vi "采配水PLC通讯.vi"() -> ()   [LabVIEW 2016, in "PLC.lvlib"]
uses:
  PLC.lvlib
  <vilib>/Plasmionique/MB Master/MB_Master/MB_Master.lvclass
  <vilib>/Plasmionique/MB Master/MB_Master_Serial/MB_Master_Serial.lvclass
  D:/Program Files (x86)/National Instruments/LabVIEW 2016/vi.lib/Plasmionique/MB Master/MB_Master/MB_Master.lvclass
  <vilib>/Plasmionique/MB Master/MB Master.lvlib
panel:
  in  "单个写入参数":T1
  in  "单个写入":bool
  in  "多个写入参数":T2
  in  "多个写入":bool
  out "元素":cluster{"命令":string, "数据":variant}[](array[cluster])
  out "待处理插入数量":i32
  out "待处理删除数量":i32
  out "队列中元素数量":i32
  in  "读状态":bool
  out "命令":string
  in  "停止":bool
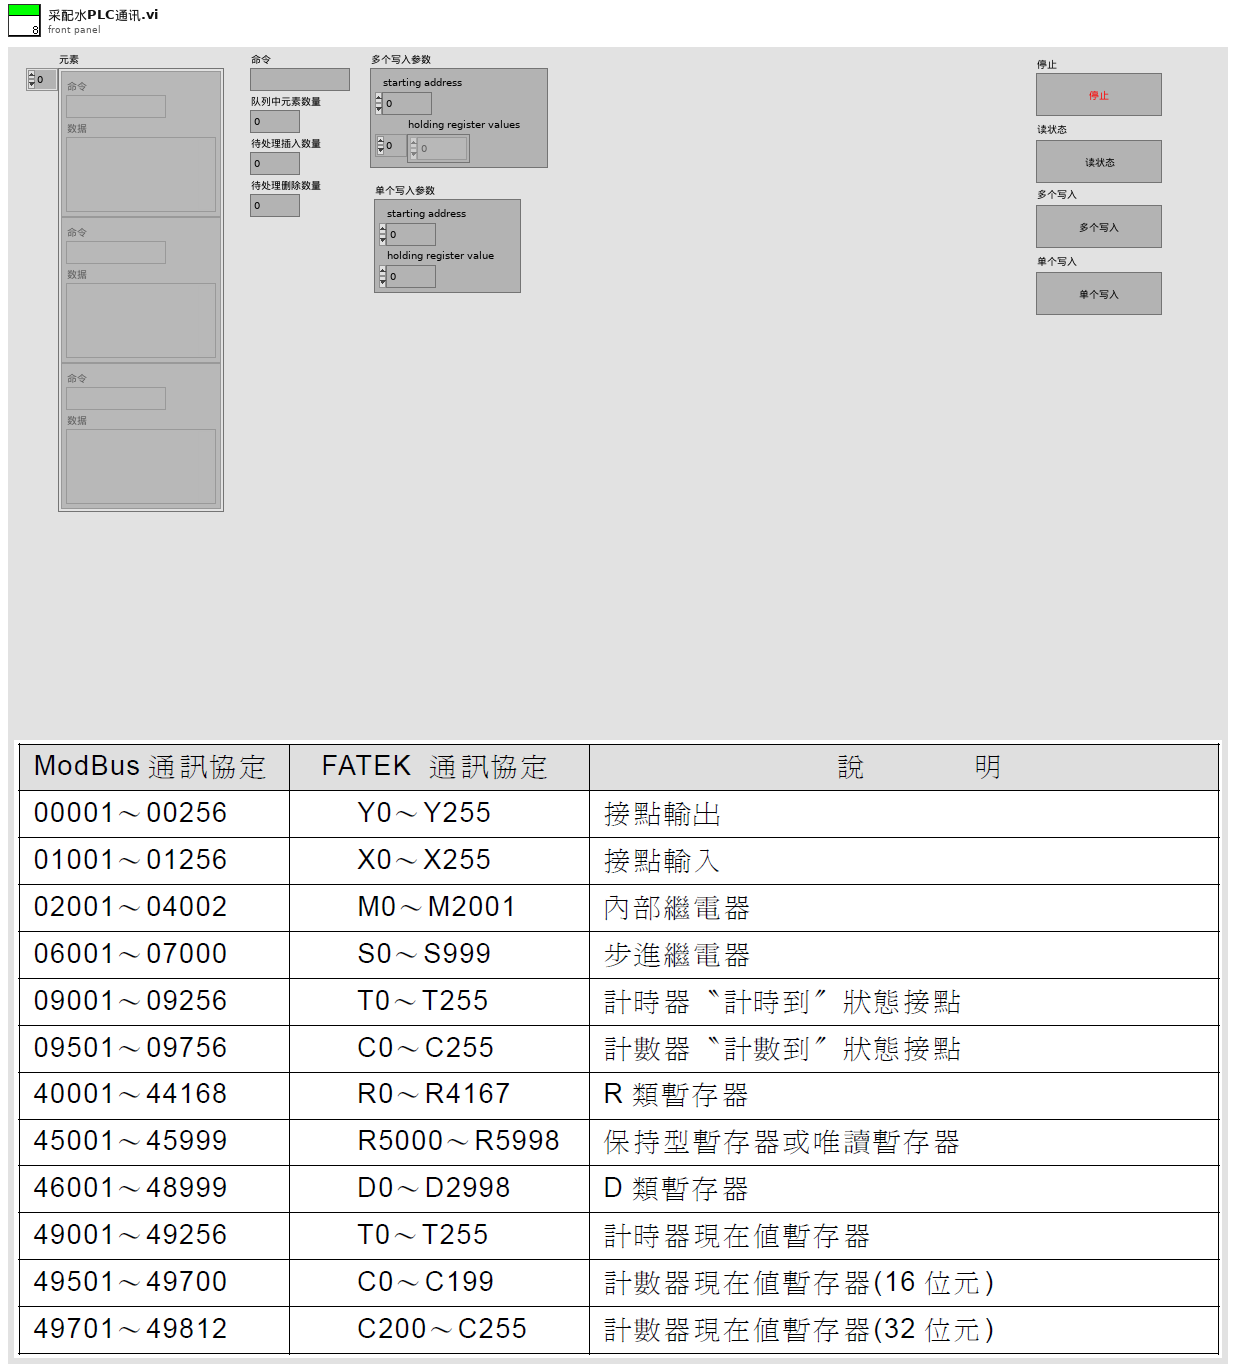
[diagram p1: front panel]
types:
  T1 = cluster{"starting address":u16, "holding register value":u16}
  T2 = cluster{"starting address":u16, "holding register values":u16[]}
  T3 = cluster{"baud rate (bps)":u32, "stop bits":u16, "parity":u16, "flow control":u16, "timeout":u32, "retries":i32}
  T4 = cluster{"starting address":u16, "coil values":bool[]}
  T5 = cluster{"Registers[0]":u16, "Registers[1]":u16, "Registers[2]":u16, "Registers[3]":u16, "Registers[4]":u16, "Registers[5]":u16, "Registers[6]":u16, "Registers[7]":u16, "Registers[8]":u16, "Registers[9]":u16, "Registers[10]":u16, "Registers[11]":u16, "Registers[12]":u16, "Registers[13]":u16, "Registers[14]":u16, "Registers[15]":u16, "Registers[16]":u16, "Registers[17]":u16, "Registers[18]":u16, "Registers[19]":u16}
  T6 = cluster{"Registers[0]":u16, "Registers[1]":u16, "Registers[2]":u16, "Registers[3]":u16, "Registers[4]":u16, "Registers[5]":u16}
  T7 = cluster{"Coils[0]":bool, "Coils[1]":bool, "Coils[2]":bool, "Coils[3]":bool, "Coils[4]":bool, "Coils[5]":bool, "Coils[6]":bool, "Coils[7]":bool, "Coils[8]":bool, "Coils[9]":bool, "Coils[10]":bool, "Coils[11]":bool, "Coils[12]":bool, "Coils[13]":bool, "Coils[14]":bool, "Coils[15]":bool}
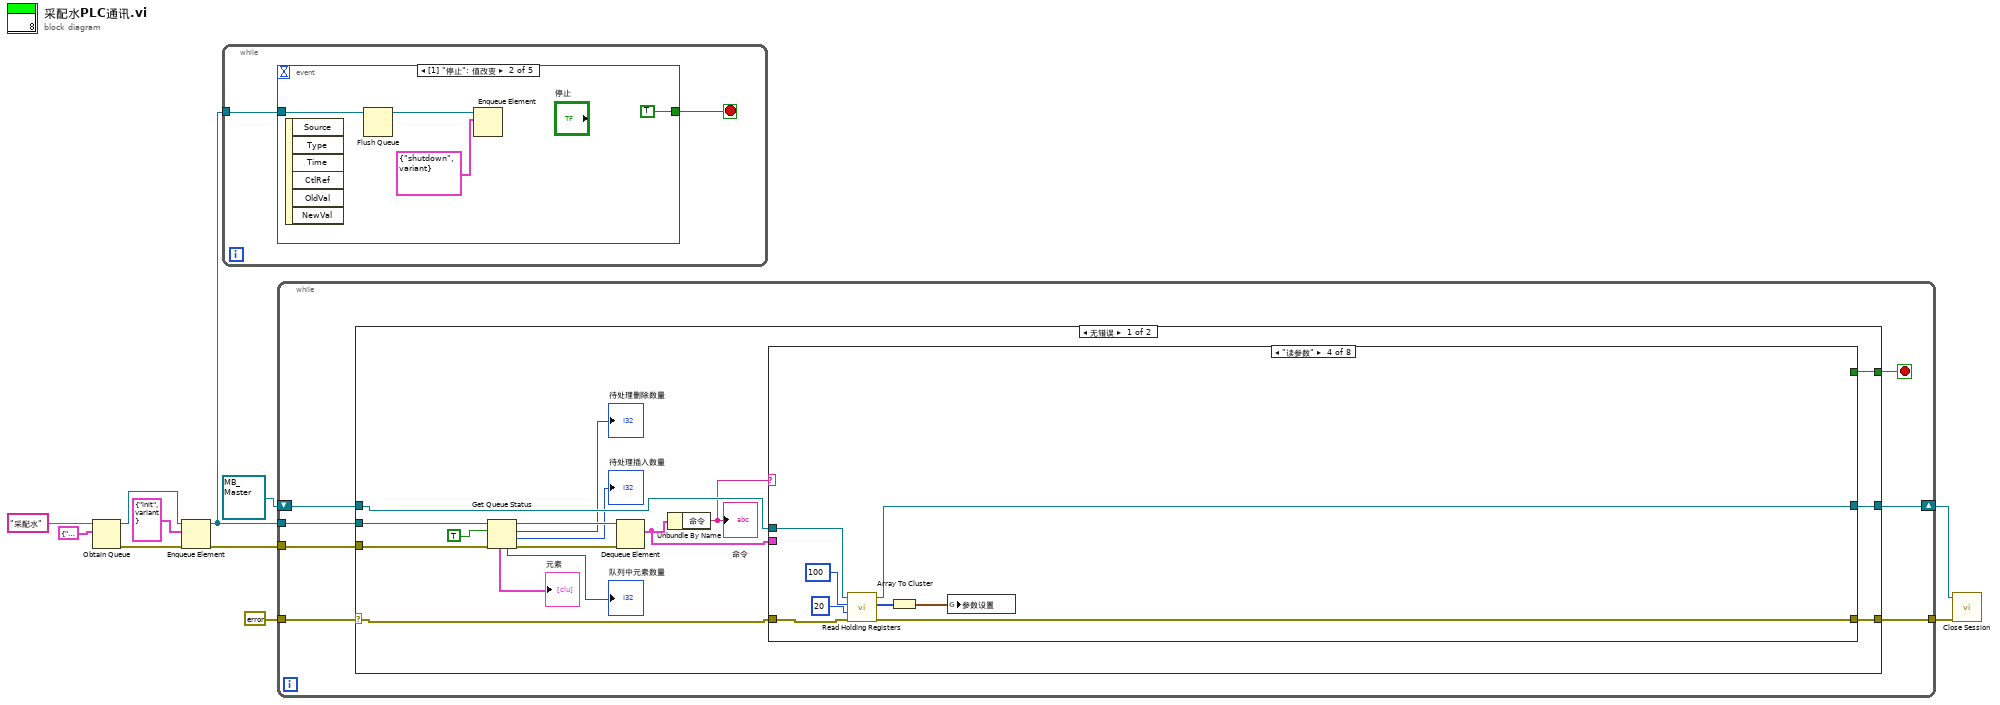
[diagram p0: block diagram]
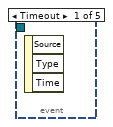
[diagram p2: hidden frame]
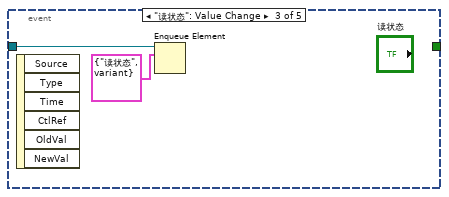
[diagram p3: hidden frame]
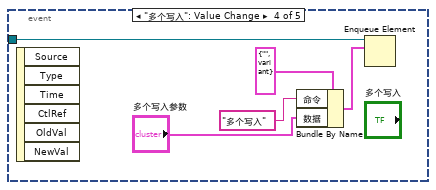
[diagram p4: hidden frame]
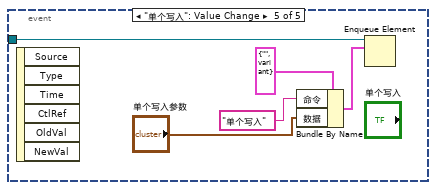
[diagram p5: hidden frame]
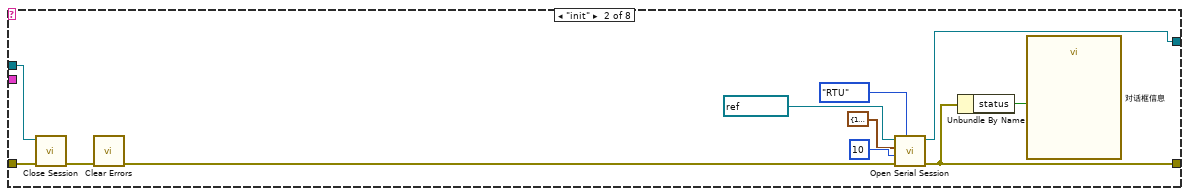
[diagram p7: hidden frame]
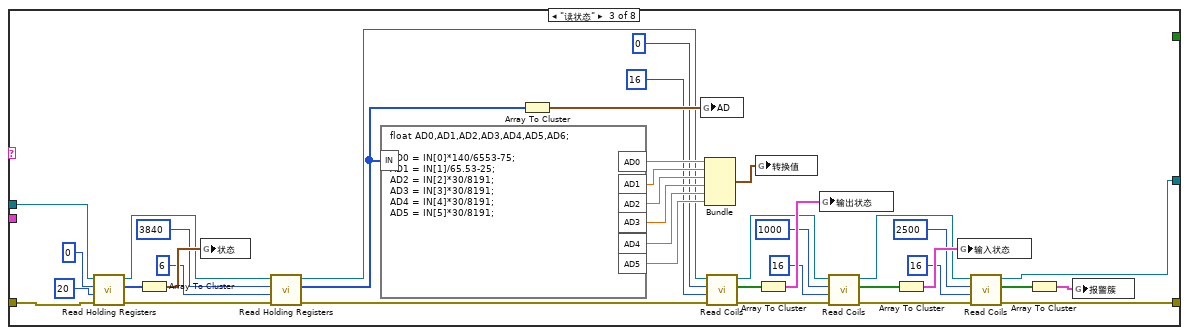
[diagram p8: hidden frame]
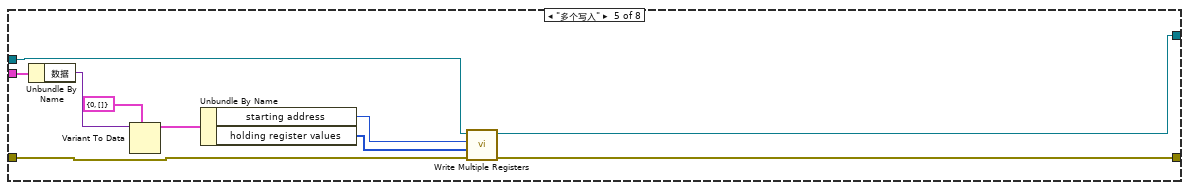
[diagram p9: hidden frame]
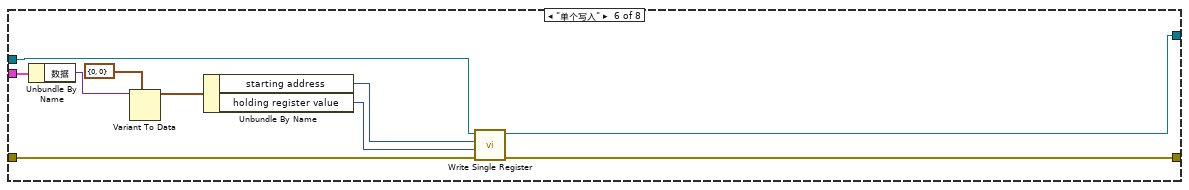
[diagram p10: hidden frame]
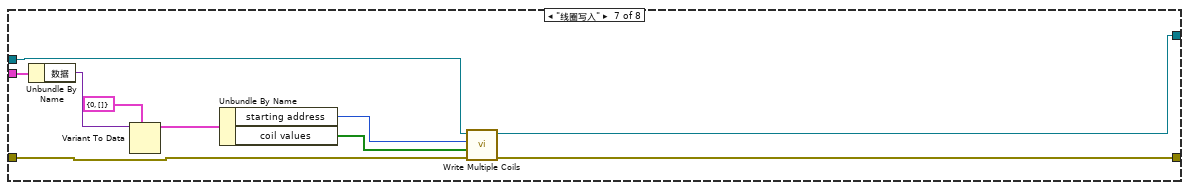
[diagram p11: hidden frame]
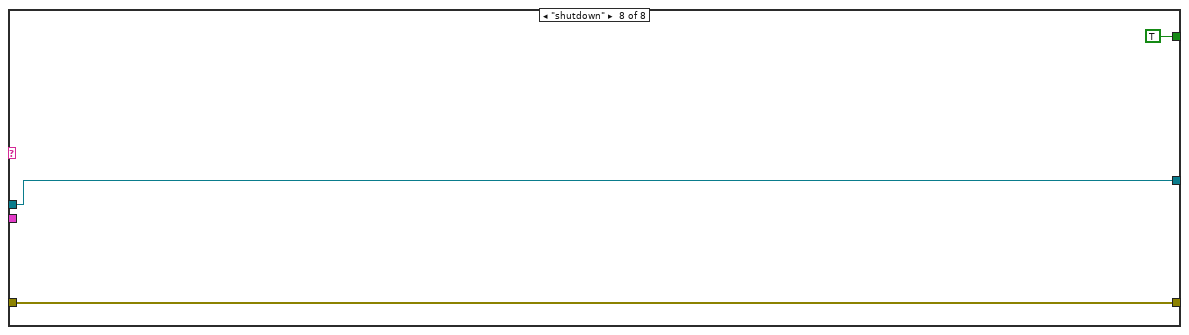
[diagram p12: hidden frame]
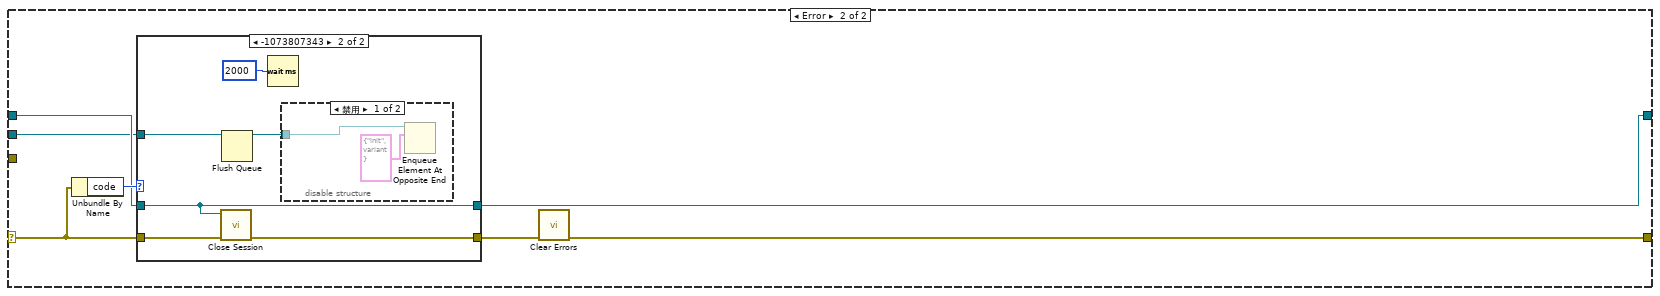
[diagram p13: hidden frame]
diagram:
  n1 = Obtain Queue(name (unnamed)="采配水" ("名称（未命名）"), element data type=cluster{"命令":string, "数据":variant} {"命令"="", "数据"=variant}) -> (queue out=w9:refnum<queue>, error out=w8:errorcluster)  [unwired: 3 in, 1 out]
  n2 = Enqueue Element(queue=w9, element=cluster{"命令":string, "数据":variant} {"命令"="init", "数据"=variant} ("元素"), error in (no error)=w8) -> (queue out=w4:refnum<queue>, error out=w6:errorcluster)  [unwired: 1 in, 1 out]
  n3 = while {
    tunnel: w4 -> [w13]
    stop <- w12 stop-if-true
    n4 = event shown="[1] \"停止\": 值改变" {
      selector: _ -> [_ _ _ _ _]
      dyn-events: _ -> [_ _ _ _ _]
      timeout: _ -> [_ _ _ _ _]
      tunnel: w13 -> [_ w16 w19 w24 w29]
      tunnel: [_ TRUE _ _ _] -> w12
      event Timeout {
        n5 = event-data() -> ()  [unwired: 1 in, 3 out]
      }
      event "停止": Value Change {
        n6 = event-data() -> ()  [unwired: 1 in, 6 out]
        n7 = Flush Queue(queue=w16) -> (queue out=w14:refnum<queue>)  [unwired: 1 in, 2 out]
        n8 = Enqueue Element(queue=w14, element=cluster{"命令":string, "数据":variant} {"命令"="shutdown", "数据"=variant} ("元素")) -> ()  [unwired: 2 in, 3 out]
      }
      event "读状态": Value Change {
        n9 = event-data() -> ()  [unwired: 1 in, 6 out]
        n10 = Enqueue Element(queue=w19, element=cluster{"命令":string, "数据":variant} {"命令"="读状态", "数据"=variant} ("元素")) -> ()  [unwired: 2 in, 3 out]
      }
      event "多个写入": Value Change {
        n11 = event-data() -> ()  [unwired: 1 in, 6 out]
        n12 = Bundle By Name(cluster=cluster{"命令":string, "数据":variant} {"命令"="", "数据"=variant} ("元素"), "命令"="多个写入", "数据"="多个写入参数") -> (w20:cluster{"命令":string, "数据":variant})
        n13 = Enqueue Element(queue=w24, element=w20) -> ()  [unwired: 2 in, 3 out]
      }
      event "单个写入": Value Change {
        n14 = event-data() -> ()  [unwired: 1 in, 6 out]
        n15 = Bundle By Name(cluster=cluster{"命令":string, "数据":variant} {"命令"="", "数据"=variant} ("元素"), "命令"="单个写入", "数据"="单个写入参数") -> (w26:cluster{"命令":string, "数据":variant})
        n16 = Enqueue Element(queue=w29, element=w26) -> ()  [unwired: 2 in, 3 out]
      }
    }
  }
  n17 = while {
    tunnel: w4 -> [w32]
    tunnel: w6 -> [w31]
    shift-right: [w36] -> w1
    shift-left: refnum<class "MB_Master.lvclass"> refnum ("MB session in") -> [w35]
    tunnel: errorcluster {"status"=FALSE, "code"=0, "source"=""} ("error out") -> [w33]
    tunnel: [w34] -> w2
    stop <- w30 stop-if-true
    n18 = case shown="无错误" w33 {
      selector: w33 -> [w49 w150]
      tunnel: [w52 w149] -> w36
      tunnel: w35 -> [w51 w151]
      tunnel: [w50 w147] -> w34
      tunnel: w32 -> [w46 w146]
      tunnel: w31 -> [w45 _]
      tunnel: [w47 _] -> w30
      frame No Error {
        n19 = Get Queue Status(queue=w46, return elements? (F)=TRUE ("返回元素？(F)"), error in (no error)=w45) -> (queue out=w44:refnum<queue>, # pending remove=→"待处理删除数量":i32, # pending insert=→"待处理插入数量":i32, error out=w43:errorcluster, # elements in queue=→"队列中元素数量":i32, elements=→"元素":cluster{"命令":string, "数据":variant}[])  [unwired: 2 out]
        n20 = Dequeue Element(queue=w44, error in (no error)=w43) -> (element=w37:cluster{"命令":string, "数据":variant})  [unwired: 1 in, 3 out]
        n21 = Unbundle By Name(w37) -> ("命令"=w48:string)
        "命令" <- w48
        n22 = case shown="\"读参数\"" w48 {
          tunnel: [w54 w58 w67 w106 w119 w129 w139 w144] -> w52
          tunnel: w51 -> [w54 w62 w89 w111 w122 w132 w142 w144]
          tunnel: [w53 w60 w66 w105 w120 w130 w140 w143] -> w50
          tunnel: w49 -> [w53 w64 w92 w110 w121 w131 w141 w143]
          tunnel: [_ _ _ _ _ _ _ TRUE] -> w47
          tunnel: w37 -> [_ _ _ _ w118 w128 w138 _]
          frame "idle", Default {
          }
          frame "init" {
            n23 = call-dynamic "Close Session.vi"("error in (no error)"=w64, "MB session in"=w62) -> ("error out"=w63:errorcluster)  [unwired: 9 in]
            n24 = call <vilib>:"Clear Errors.vi"("error in (no error)"=w63) -> ("error out"=w61:errorcluster)  [unwired: 5 in, 1 out]
            n25 = call <vilib>:"Open Serial Session.vi"("Mode (RTU)"=enum16{"RTU", "ASCII"}."RTU", "Error in"=w61, "Slave ID"=u8 10, "Serial Config"=T3 {"baud rate (bps)"=115200, "stop bits"=10, "parity"=0, "flow control"=0, "timeout"=1000, "retries"=1}, "VISA Resource"=refnum<visa-resource-name> "COM2" ("VISA resource name")) -> ("Error out"=w60:errorcluster, "MB_Serial session"=w58:refnum<class "MB_Master_Serial.lvclass">)  [unwired: 5 in]
            n26 = Unbundle By Name(w60) -> ("status"=w65:bool)
            n27 = call "对话框信息"("Enable"=w65) -> ()  [unwired: 9 in, 2 out]
          }
          frame "读状态" {
            n28 = call <vilib>:"Read Holding Registers.vi"("error in (no error)"=w92, "quantity"=u16 20 ("number of holding registers"), "starting address"=u16 0, "MB session in"=w89) -> ("error out"=w85:errorcluster, "Registers"=w88:u16[], "MB session out"=w87:refnum<class "MB_Master.lvclass">)  [unwired: 5 in]
            n29 = Array To Cluster(array=w88) -> (cluster=w94:T5)
            n30 = global write "采配水全局变量.vi" "状态"(w94) -> ()
            n31 = call <vilib>:"Read Holding Registers.vi"("error in (no error)"=w85, "quantity"=u16 6 ("number of holding registers"), "starting address"=u16 3840, "MB session in"=w87) -> ("error out"=w81:errorcluster, "Registers"=w86:u16[], "MB session out"=w82:refnum<class "MB_Master.lvclass">)  [unwired: 5 in]
            n32 = formula code="float AD0,AD1,AD2,AD3,AD4,AD5,AD6;\n\nAD0 = IN[0]*140/6553-75;\nAD1 = IN[1]/65.53-25;\nAD2 = IN[2]*30/8191;\nAD3 = IN[3]*30/8191;\nAD4 = IN[4]*30/8191;\nAD5 = IN[5]*30/8191;"("IN"=w86) -> ("AD0"=w100:dbl, "AD1"=w99:dbl, "AD2"=w98:dbl, "AD3"=w97:dbl, "AD4"=w96:dbl, "AD5"=w95:dbl)
            n33 = Array To Cluster(array=w86) -> (cluster=w102:T6)
            n34 = global write "采配水全局变量.vi" "AD"(w102) -> ()
            n35 = Bundle(w100, w99, w98, w97, w96, w95) -> (w101:cluster{dbl, dbl, dbl, dbl, dbl, dbl})  [unwired: 1 in]
            n36 = call <vilib>:"Read Coils.vi"("error in (no error)"=w81, "quantity"=u16 16 ("number of coils"), "starting address"=u16 0, "MB session in"=w82) -> ("error out"=w76:errorcluster, "Coils"=w78:bool[], "MB session out"=w77:refnum<class "MB_Master.lvclass">)  [unwired: 5 in]
            n37 = global write "采配水全局变量.vi" "转换值"(w101) -> ()
            n38 = Array To Cluster(array=w78) -> (cluster=w103:T7)
            n39 = global write "采配水全局变量.vi" "输出状态"(w103) -> ()
            n40 = call <vilib>:"Read Coils.vi"("error in (no error)"=w76, "quantity"=u16 16 ("number of coils"), "starting address"=u16 1000, "MB session in"=w77) -> ("error out"=w72:errorcluster, "Coils"=w71:bool[], "MB session out"=w73:refnum<class "MB_Master.lvclass">)  [unwired: 5 in]
            n41 = Array To Cluster(array=w71) -> (cluster=w104:T7)
            n42 = global write "采配水全局变量.vi" "输入状态"(w104) -> ()
            n43 = call <vilib>:"Read Coils.vi"("error in (no error)"=w72, "quantity"=u16 16 ("number of coils"), "starting address"=u16 2500, "MB session in"=w73) -> ("error out"=w66:errorcluster, "Coils"=w68:bool[], "MB session out"=w67:refnum<class "MB_Master.lvclass">)  [unwired: 5 in]
            n44 = Array To Cluster(array=w68) -> (cluster=w93:T7)
            n45 = global write "采配水全局变量.vi" "报警簇"(w93) -> ()
          }
          frame "读参数" {
            n46 = call <vilib>:"Read Holding Registers.vi"("error in (no error)"=w110, "quantity"=u16 20 ("number of holding registers"), "starting address"=u16 100, "MB session in"=w111) -> ("error out"=w105:errorcluster, "Registers"=w107:u16[], "MB session out"=w106:refnum<class "MB_Master.lvclass">)  [unwired: 5 in]
            n47 = Array To Cluster(array=w107) -> (cluster=w112:T5)
            n48 = global write "采配水全局变量.vi" "参数设置"(w112) -> ()
          }
          frame "多个写入" {
            n49 = Unbundle By Name(w118) -> ("数据"=w117:variant)
            n50 = Variant To Data(type=T2 {"starting address"=0, "holding register values"=[]}, Variant=w117) -> (data=w115:T2)  [unwired: 1 in, 1 out]
            n51 = Unbundle By Name(w115) -> ("starting address"=w114:u16, "holding register values"=w113:u16[])
            n52 = call <vilib>:"Write Multiple Registers.vi"("error in (no error)"=w121, "values"=w113, "starting address"=w114, "MB session in"=w122) -> ("error out"=w120:errorcluster, "MB session out"=w119:refnum<class "MB_Master.lvclass">)  [unwired: 6 in]
          }
          frame "单个写入" {
            n53 = Unbundle By Name(w128) -> ("数据"=w127:variant)
            n54 = Variant To Data(type=T1 {"starting address"=0, "holding register value"=0}, Variant=w127) -> (data=w125:T1)  [unwired: 1 in, 1 out]
            n55 = Unbundle By Name(w125) -> ("starting address"=w124:u16, "holding register value"=w123:u16)
            n56 = call <vilib>:"Write Single Register.vi"("error in (no error)"=w131, "value"=w123, "address"=w124, "MB session in"=w132) -> ("error out"=w130:errorcluster, "MB session out"=w129:refnum<class "MB_Master.lvclass">)  [unwired: 6 in]
          }
          frame "线圈写入" {
            n57 = Unbundle By Name(w138) -> ("数据"=w137:variant)
            n58 = Variant To Data(type=T4 {"starting address"=0, "coil values"=[]}, Variant=w137) -> (data=w135:T4)  [unwired: 1 in, 1 out]
            n59 = Unbundle By Name(w135) -> ("starting address"=w134:u16, "coil values"=w133:bool[])
            n60 = call <vilib>:"Write Multiple Coils.vi"("error in (no error)"=w141, "values"=w133, "starting address"=w134, "MB session in"=w142) -> ("error out"=w140:errorcluster, "MB session out"=w139:refnum<class "MB_Master.lvclass">)  [unwired: 6 in]
          }
          frame "shutdown" {
          }
        }
      }
      frame Error {
        n61 = Unbundle By Name(w150) -> ("code"=w152:i32)
        n62 = case shown="-1073807343" w152 {
          tunnel: w151 -> [w154 w158]
          tunnel: w150 -> [w153 w160]
          tunnel: [w153 w159] -> w148
          tunnel: [w154 w158] -> w149
          tunnel: w146 -> [_ w157]
          frame Default {
          }
          frame -1073807343 {
            n63 = call-dynamic "Close Session.vi"("error in (no error)"=w160, "MB session in"=w158) -> ("error out"=w159:errorcluster)  [unwired: 9 in]
            n64 = Flush Queue(queue=w157) -> (queue out=w156:refnum<queue>)  [unwired: 1 in, 2 out]
            n65 = Wait (ms)(milliseconds to wait=u32 2000 ("等待时间（毫秒）")) -> ()  [unwired: 1 out]
            n66 = disable-structure shown="禁用" {
              disable-tunnel: w156 -> [w161 _]
              frame Disabled {
                n67 = Enqueue Element At Opposite End(queue=w161, element=cluster{"命令":string, "数据":variant} {"命令"="init", "数据"=variant} ("元素")) -> ()  [unwired: 2 in, 3 out]
              }
              frame Enabled {
              }
            }
          }
        }
        n68 = call <vilib>:"Clear Errors.vi"("error in (no error)"=w148) -> ("error out"=w147:errorcluster)  [unwired: 5 in, 1 out]
      }
    }
  }
  n69 = call-dynamic "Close Session.vi"("error in (no error)"=w2, "MB session in"=w1) -> ()  [unwired: 9 in, 1 out]
